vi "Quick Start - Streaming - Write.vi"() -> ()   [LabVIEW 2020]
uses:
  Nominal Client/Nominal Client.lvclass/Nominal Client.ctl
  68912467-c1c9-4a94-a3ad-dccbebf4617c.vi
  d588a604-dc97-41f6-8cdf-6e6429fb216e.vi
  8bc873d6-11f2-47b8-afa9-2ee06eb45ce7.vi
  d588a604-dc97-41f6-8cdf-6e6429fb216e.vi/028fdd67-09da-40c6-8995-0c4bd62a0b31.vi
  <vilib>/JDP Science/JSONtext/Make JSON Object.vi
  d588a604-dc97-41f6-8cdf-6e6429fb216e.vi/c2a1aca9-ea5a-4b2a-8072-18de54756c53.vi
  <vilib>/JDP Science/JSONtext/Make JSON Array.vi
  d588a604-dc97-41f6-8cdf-6e6429fb216e.vi/2c8a2fb0-06af-4bda-9dcc-d72a85547e70.vi
  Nominal Client/private_data.set.vi
  <vilib>/LabVIEW Open Source Project/Epoch Date & Time/epoch.UNIX/Epoch.UNIX.lvclass
  C:/Program Files/National Instruments/LabVIEW 2020/vi.lib/LabVIEW Open Source Project/Epoch Date & Time/epoch/Epoch.lvclass
  <vilib>/Utility/file.llb/Application Directory.vi
  <vilib>/Utility/error.llb/Error Cluster From Error Code.vi
  submodules/reqwest-labview/lv-src/reqwest/create.vi
  <vilib>/LabVIEW Open Source Project/Epoch Date & Time/Get Epoch Time.vi
  Nominal Client/nominal_channel_writer.write_batches.path.vi
  nominal types/properties/create.from_cluster_pairs.vi
  <vilib>/JDP Science/JSONtext/Variant to JSON Text.vi
  <vilib>/JDP Science/JSONtext/support/Format JSON Object.vi
  <vilib>/JDP Science/JSONtext/support/Format JSON Array Text.vi
  Nominal Client/http.post.vi
  Nominal Client/Nominal Client.lvclass
  nominal types/workspace/workspace.lvclass
  submodules/reqwest-labview/lv-src/reqwest/reqwest.lvclass
  <vilib>/JDP Science/JSONtext/LVClass Serializer/JSONtext LVClass Serializer.lvclass
  nominal types/properties/properties.lvclass
panel:
  in  "API Token":string
  in  "Data Source RID":string
  in  "Stop":bool
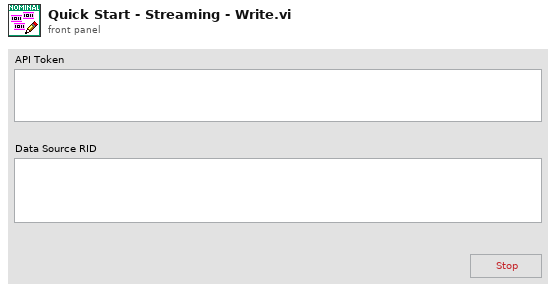
[diagram p1: front panel]
types:
  T1 = cluster{"channel":string, "current time":timestamp, "data":dbl}
  T2 = cluster{"[0]":refnum<queue>, "[1]":refnum<queue>, "[2]":refnum<queue>}
  T3 = cluster{"channel":string, "current time":timestamp, "data":dbl}[]
  T4 = cluster{"UNIX Timestamp":cluster{"Seconds":i64, "Nanoseconds":i64}, "data":dbl}
  T5 = cluster{"channel":string, cluster{"UNIX Timestamp":cluster{"Seconds":i64, "Nanoseconds":i64}, "data":dbl}[]}
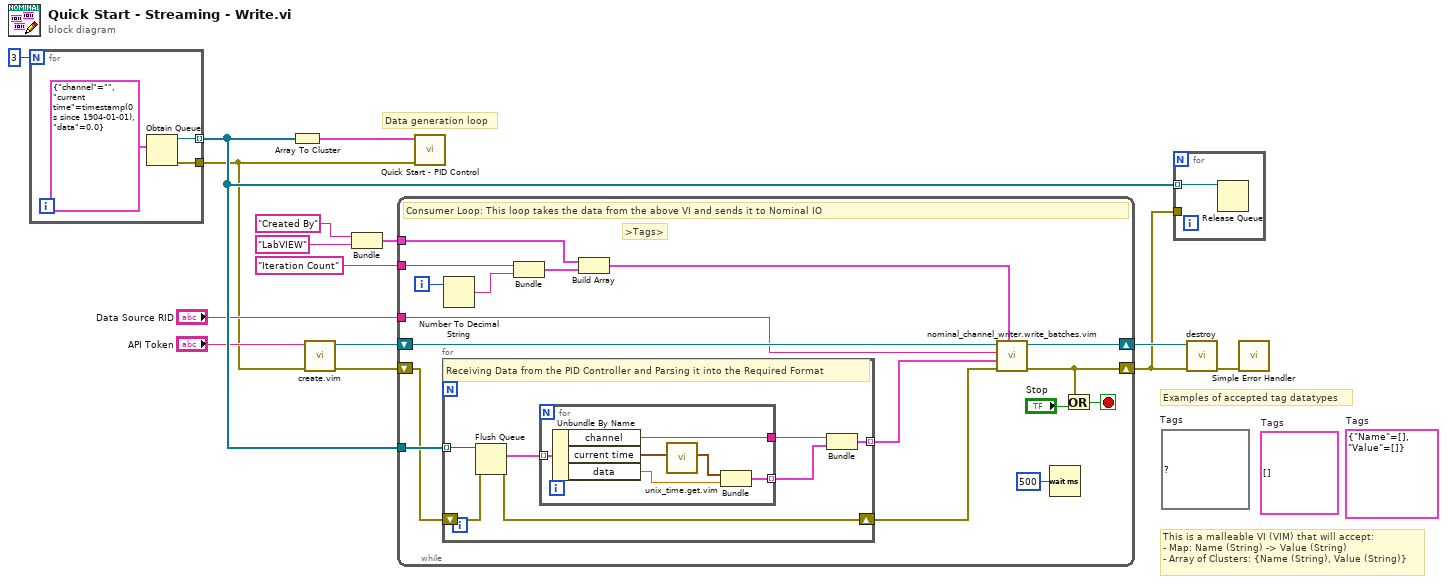
[diagram p0: block diagram]
diagram:
  (unwired) cluster{"Name":string[], "Value":string[]} {"Name"=[], "Value"=[]}  # Tags
  (unwired) cluster{"Name":string, "Value":string}[] []  # Tags
  (unwired) map{string, string} {}  # Tags
  # "Examples of accepted tag datatypes"
  # "This is a malleable VI (VIM) that will accept:\n- Map: Name (String) -> Value (String)\n- Array of Clusters: {Name (String), Value (String)}"
  # "Data generation loop"
  n1 = for {
    N: 3 -> [_]
    tunnel: [w17] -> w10 mode=indexing
    tunnel: [w16] -> w5
    n2 = Obtain Queue(element data type=T1 {"channel"="", "current time"=timestamp(0 s since 1904-01-01), "data"=0.0}) -> (queue out=w17:refnum<queue>, error out=w16:errorcluster)  [unwired: 4 in, 1 out]
  }
  n3 = Array To Cluster(array=w10) -> (cluster=w6:T2)
  n4 = call "create.vim"("error in"=w5, "API Token (string or path)"="API Token") -> ("error out"=w13:errorcluster, "Nominal Client"=w14:refnum<class "Nominal Client.lvclass">)  [unwired: 8 in]
  n5 = Bundle("Created By", "LabVIEW") -> (w1:cluster{string, string})  [unwired: 1 in]
  n6 = while {
    tunnel: w10 -> [w32]
    shift-right: [w22] -> w9
    shift-left: w13 -> [w31]
    shift-right: [w21] -> w15
    shift-left: w14 -> [w25]
    tunnel: "Data Source RID" -> [w24]
    tunnel: "Iteration Count" -> [w28]
    tunnel: w1 -> [w27]
    i -> [w30]
    stop <- w34 stop-if-true
    # ">Tags>"
    # "Consumer Loop: This loop takes the data from the above VI and sends it to Nominal IO"
    n7 = for {
      tunnel: w32 -> [w42] mode=indexing
      tunnel: [w38] -> w19 mode=indexing
      shift-right: [w36] -> w23
      shift-left: w31 -> [w37]
      # "Receiving Data from the PID Controller and Parsing it into the Required Format"
      n8 = Flush Queue(queue=w42, error in (no error)=w37) -> (remaining elements=w41:T3, error out=w36:errorcluster)  [unwired: 1 out]
      n9 = for {
        tunnel: w41 -> [w48] mode=indexing
        tunnel: [w44] -> w39 mode=indexing
        tunnel: [w43] -> w40
        n10 = Unbundle By Name(w48) -> ("channel"=w43:string, "current time"=w47:timestamp, "data"=w45:dbl)
        n11 = call "unix_time.get.vim"("Time Stamp (empty: now) [single or array]"=w47) -> ("UNIX Timestamp"=w46:cluster{"Seconds":i64, "Nanoseconds":i64})  [unwired: 10 in]
        n12 = Bundle("UNIX Timestamp"=w46, "data"=w45) -> (w44:T4)  [unwired: 1 in]
      }
      n13 = Bundle("channel"=w40, w39) -> (w38:T5)  [unwired: 1 in]
    }
    n14 = Number To Decimal String(number=w30) -> (decimal integer string=w29:string)  [unwired: 1 in]
    n15 = Bundle(w28, w29) -> (w26:cluster{string, string})  [unwired: 1 in]
    n16 = Build Array(w27, w26) -> (w20:cluster{string, string}[])
    n17 = call "nominal_channel_writer.write_batches.vim"("Tags"=w20, "error in"=w23, "batches"=w19, "Data Source RID"=w24, "Nominal Client in"=w25) -> ("error out"=w22:errorcluster, "Nominal Client out"=w21:refnum<class "Nominal Client.lvclass">)  [unwired: 4 in, 1 out]
    n18 = Wait (ms)(milliseconds to wait=u32 500) -> ()  [unwired: 1 out]
    n19 = Or(x=w22, y="Stop") -> (x .or. y?=w34:bool)
  }
  n20 = call "Quick Start - PID Control.vi"("error in (no error)"=w5, "Data"=w6) -> ()  [unwired: 10 in]
  n21 = for {
    tunnel: w10 -> [w49] mode=indexing
    tunnel: w9 -> [_]
    n22 = Release Queue(queue=w49) -> ()  [unwired: 2 in, 3 out]
  }
  n23 = call "destroy.vi"("error in"=w9, "Nominal Client"=w15) -> ("error out"=w12:errorcluster)  [unwired: 9 in]
  n24 = call <vilib>:"Simple Error Handler.vi"("error in (no error)"=w12) -> ()  [unwired: 4 in, 5 out]
